vi "PMAC3000 get peak.vi"(8 "error in (no error)":errorcluster, 11 "Handle":i32) -> (0 "error out":errorcluster, 1 "peakInfo":string, 2 "peaknumber":i32, 3 "LivePeak":sgl)   [LabVIEW 2018]
uses:
  ftd2xx.dll
panel:
  # "input"
  # "output"
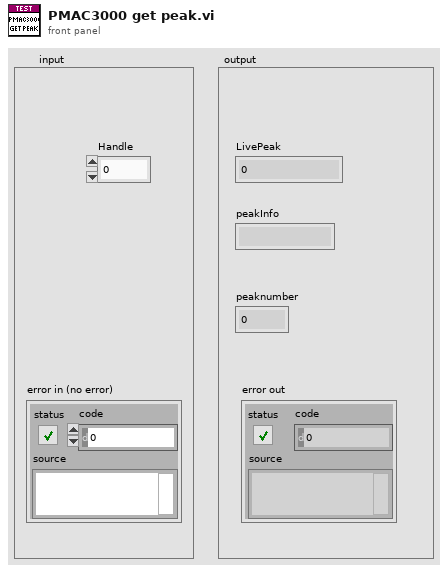
[diagram p1: front panel]
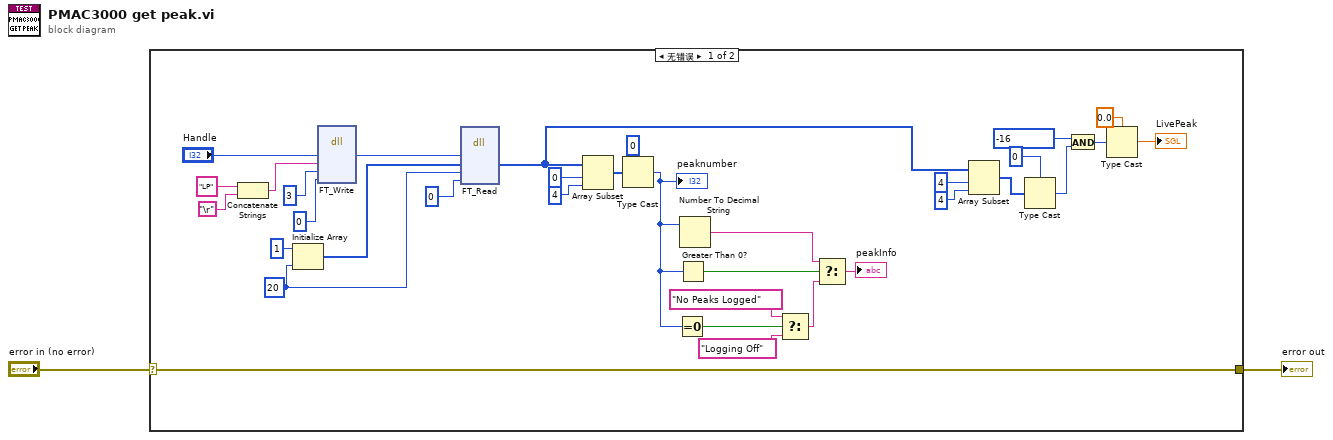
[diagram p0: block diagram]
diagram:
  n1 = case shown="无错误" "error in (no error)" {
    selector: "error in (no error)" -> [w3 w37]
    tunnel: [w3 w37] -> w1
    frame No Error {
      w25 = 20 ("dimension size")
      n2 = Concatenate Strings("LP" ("string"), "\r") -> (w17:string)
      n3 = Initialize Array(u8 1 ("element"), w25) -> (w24:u8[])
      n4 = dll-call lib="C:/Labview Code/04.SubVI's/Others VI's/FTD2XX.dll" fn="FT_Write"("Handle"="Handle", "Buffer"=w17, "BytesToWrite"=3, "BytesWritten"=0) -> ("Handle"=w21:i32)  [unwired: 7 in, 2 out]
      n5 = dll-call lib="C:/Labview Code/04.SubVI's/Others VI's/FTD2XX.dll" fn="FT_Read"("Handle"=w21, "Buffer"=w24, "BytesToRead"=w25, "BytesReturned"=0) -> ("Buffer"=w6:u8[])  [unwired: 7 in, 2 out]
      n6 = Array Subset(array=w6, index=0, length=4) -> (w28:u8[])
      n7 = Type Cast(type=0, x=w28) -> (*(type *) &x=w32:i32)
      "peaknumber" <- w32
      n8 = Equal To 0?(x=w32) -> (x = 0?=w33:bool)
      n9 = Greater Than 0?(x=w32) -> (x > 0?=w30:bool)
      n10 = Number To Decimal String(number=w32) -> (decimal integer string=w31:string)  [unwired: 1 in]
      n11 = Select(t="No Peaks Logged", s=w33, f="Logging Off") -> (s? t:f=w36:string)
      n12 = Select(t=w31, s=w30, f=w36) -> (s? t:f=→"peakInfo":string)
      n13 = Array Subset(array=w6, index=4, length=4) -> (w9:u8[])
      n14 = Type Cast(type=0, x=w9) -> (*(type *) &x=w14:i32)
      n15 = And(x=-16, y=w14) -> (x .and. y?=w12:i32)
      n16 = Type Cast(type=sgl 0.0, x=w12) -> (*(type *) &x=→"LivePeak":sgl)
    }
    frame Error {
    }
  }
  "error out" <- w1
